vi "Scan start (SubVI).vi"(0 "VISA Refnum in":refnum<visa-resource-name>="COM7", 1 "end_x":dbl, 2 "end_y":dbl, 3 "sp_x":dbl, 4 "sp_y":dbl, 5 "error in":errorcluster, 8 "Режим\nсканирования":enum32{"Ampl", "Phase"}(ring), 9 "step_x":u32, 10 "pos_xy":cluster{"pos_x":dbl, "pos_y":dbl} caption="Позиция 2D, мм", 11 "step_y":u32) -> (14 "VISA resource name out":refnum<visa-resource-name>, 16 "set_pos_xy":cluster{"pos_x":dbl, "pos_y":dbl} caption="Set pos 2D, мм", 19 "error out":errorcluster)   [LabVIEW 2018]
uses:
  GlobalStop.vi
panel:
  out "err":errorcluster
  in  "Average":u8=5 caption="Число усреднений\nАЦП" min=1 max=9
  in  "Smooth":bool=TRUE caption="Аппроксимировать\nзначения с АЦП"
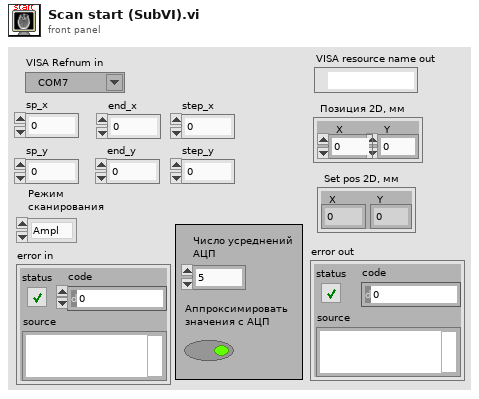
[diagram p1: front panel]
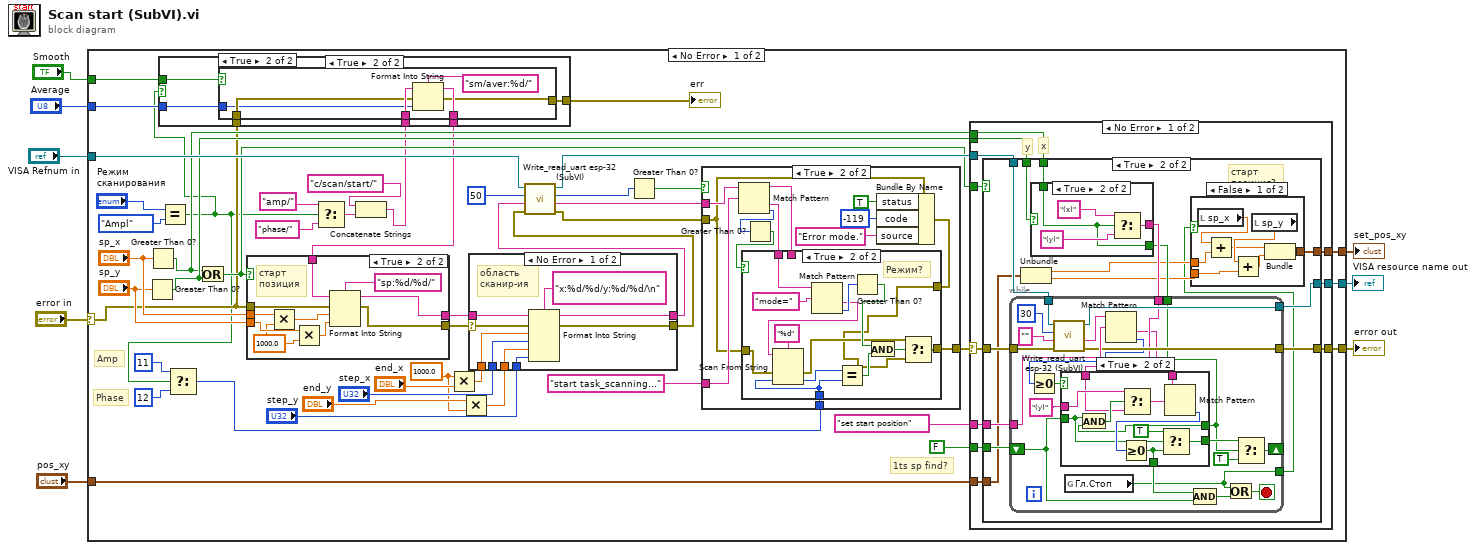
[diagram p0: block diagram]
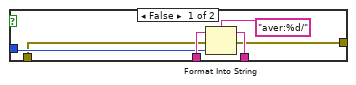
[diagram p3: hidden frame]
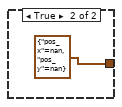
[diagram p5: hidden frame]
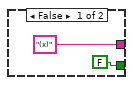
[diagram p6: hidden frame]
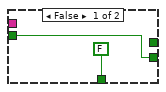
[diagram p7: hidden frame]
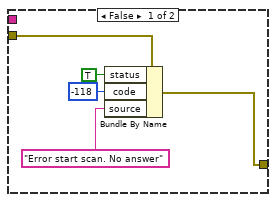
[diagram p9: hidden frame]
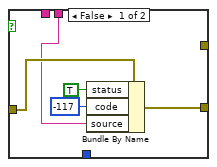
[diagram p10: hidden frame]
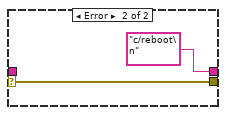
[diagram p11: hidden frame]
diagram:
  n1 = case shown="No Error" "error in" {
    selector: "error in" -> [w11 w219]
    tunnel: [w24 w219] -> w7
    tunnel: [w26 w218] -> w6
    tunnel: "VISA Refnum in" -> [w25 w218]
    tunnel: "pos_xy" -> [w17 w217]
    tunnel: [w16 w217] -> w3
    tunnel: "Smooth" -> [w15 _]
    tunnel: "Average" -> [w12 _]
    frame No Error {
      w29 = 1000.0
      # "1ts sp find?"
      # "Phase"
      # "Amp"
      n2 = Greater Than 0?(x="sp_y") -> (x > 0?=w21:bool)
      n3 = Greater Than 0?(x="sp_x") -> (x > 0?=w20:bool)
      n4 = Equal?(x="Режим\nсканирования", y=enum32{"Ampl", "Phase"}."Ampl") -> (x = y?=w9:bool)
      n5 = Select(t=u8 11, s=w9, f=u8 12) -> (s? t:f=w33:u8)
      n6 = Or(x=w20, y=w21) -> (x .or. y?=w23:bool)
      n7 = Select(t="amp/" ("initial string"), s=w9, f="phase/" ("initial string")) -> (s? t:f=w54:string)
      n8 = Concatenate Strings("c/scan/start/" ("initial string"), w54) -> (w14:string)
      n9 = case shown="True" w9 {
        tunnel: w15 -> [_ w63]
        tunnel: w14 -> [w57 w62]
        tunnel: [w57 w61] -> w13
        tunnel: w12 -> [_ w60]
        tunnel: w11 -> [w56 w59]
        tunnel: [w56 w58] -> w10
        frame False {
        }
        frame True {
          n10 = case shown="True" w63 {
            tunnel: w62 -> [w69 w73]
            tunnel: [w68 w74] -> w61
            tunnel: w60 -> [w66 w71]
            tunnel: w59 -> [w65 w72]
            tunnel: [w64 w70] -> w58
            frame False {
              n11 = Format Into String(format string="aver:%d/" ("initial string"), initial string=w69, error in=w65, w66) -> (resulting string=w68:string, error out=w64:errorcluster)
            }
            frame True {
              n12 = Format Into String(format string="sm/aver:%d/" ("initial string"), initial string=w73, error in=w72, w71) -> (resulting string=w74:string, error out=w70:errorcluster)
            }
          }
        }
      }
      "err" <- w10
      n13 = case shown="True" w23 {
        tunnel: w13 -> [w205 w216]
        tunnel: "sp_x" -> [_ w210]
        tunnel: "sp_y" -> [_ w211]
        tunnel: w11 -> [w206 w214]
        tunnel: [w206 w212] -> w47
        tunnel: [w205 w213] -> w46
        frame False {
        }
        frame True {
          w209 = 1000.0
          # "старт\nпозиция"
          n14 = Multiply(x=w210, y=w209) -> (x*y=w207:dbl)
          n15 = Multiply(x=w211, y=w209) -> (x*y=w208:dbl)
          n16 = Format Into String(format string="sp:%d/%d/", initial string=w216, error in=w214, w207, w208) -> (resulting string=w213:string, error out=w212:errorcluster)
        }
      }
      n17 = Multiply(x=w29, y="end_x") -> (x*y=w31:dbl)
      n18 = Multiply(x="end_y", y=w29) -> (x*y=w28:dbl)
      n19 = case shown="No Error" w47 {
        selector: w47 -> [w201 w204]
        tunnel: w46 -> [w202 _]
        tunnel: w31 -> [w200 _]
        tunnel: "step_x" -> [w198 _]
        tunnel: w28 -> [w197 _]
        tunnel: "step_y" -> [w196 _]
        tunnel: [w195 w204] -> w42
        tunnel: [w194 "c/reboot\n"] -> w41
        frame No Error {
          # "область\nсканир-ия"
          n20 = Format Into String(format string="x:%d/%d/y:%d/%d/\n", initial string=w202, error in=w201, w200, w198, w197, w196) -> (resulting string=w194:string, error out=w195:errorcluster)
        }
        frame Error {
        }
      }
      n21 = call "Write_read_uart esp-32 (SubVI).vi"("error in (no error)"=w42, "write buffer"=w41, "milliseconds to wait"=u32 50, "VISA Refnum in"=w25) -> ("error out 4"=w37:errorcluster, "read buffer"=w40:string, "read bite"=w39:u32, "VISA resource name out"=w27:refnum<visa-resource-name>)
      n22 = Greater Than 0?(x=w39) -> (x > 0?=w38:bool)
      n23 = case shown="True" w38 {
        tunnel: w40 -> [_ w174]
        tunnel: w37 -> [w159 w166]
        tunnel: "start task_scanning..." -> [_ w173]
        tunnel: w33 -> [_ w169]
        tunnel: [w158 w164] -> w18
        frame False {
          n24 = Bundle By Name(cluster=w159, "status"=TRUE, "code"=i16 -118, "source"="Error start scan. No answer") -> (w158:errorcluster)
        }
        frame True {
          n25 = Match Pattern(string=w174, regular expression=w173) -> (before substring=w162:string, after substring=w170:string, offset past match=w172:i32)  [unwired: 1 in, 1 out]
          n26 = Greater Than 0?(x=w172) -> (x > 0?=w171:bool)
          n27 = Bundle By Name(cluster=w166, "status"=TRUE, "code"=i16 -119, "source"="Error mode.") -> (w165:errorcluster)
          n28 = case shown="True" w171 {
            tunnel: w170 -> [_ w193]
            tunnel: w166 -> [w178 w188]
            tunnel: w169 -> [_ w187]
            tunnel: w165 -> [_ w181]
            tunnel: [w177 w180] -> w164
            tunnel: w162 -> [w175 _]
            frame False {
              n29 = Bundle By Name(cluster=w178, "status"=TRUE, "code"=i16 -117, "source"=w175) -> (w177:errorcluster)
            }
            frame True {
              # "Режим?"
              n30 = Match Pattern(string=w193, regular expression="mode=") -> (after substring=w189:string, offset past match=w191:i32)  [unwired: 1 in, 2 out]
              n31 = Scan From String(format string="%d", input string=w189, error in=w188, default 1=w187) -> (error out=w182:errorcluster, output 1=w186:u8)  [unwired: 1 in, 2 out]
              n32 = Equal?(x=w186, y=w187) -> (x = y?=w184:bool)
              n33 = Greater Than 0?(x=w191) -> (x > 0?=w185:bool)
              n34 = And(x=w185, y=w184) -> (x .and. y?=w183:bool)
              n35 = Select(t=w182, s=w183, f=w181) -> (s? t:f=w180:errorcluster)
            }
          }
        }
      }
      n36 = case shown="No Error" w18 {
        selector: w18 -> [w78 w155]
        tunnel: w27 -> [w86 w156]
        tunnel: [w85 w156] -> w26
        tunnel: [w84 w155] -> w24
        tunnel: w23 -> [w83 _]
        tunnel: "set start position" -> [w82 _]
        tunnel: w21 -> [w81 _]
        tunnel: w20 -> [w80 _]
        tunnel: FALSE -> [w79 _]
        tunnel: w17 -> [w77 w154]
        tunnel: [w76 w154] -> w16
        frame No Error {
          # "x"
          # "y"
          n37 = case shown="True" w83 {
            tunnel: w86 -> [w89 w104]
            tunnel: [w89 w103] -> w85
            tunnel: w78 -> [w88 w102]
            tunnel: [w88 w101] -> w84
            tunnel: w82 -> [_ w100]
            tunnel: w81 -> [_ w99]
            tunnel: w80 -> [_ w98]
            tunnel: w79 -> [_ w96]
            tunnel: w77 -> [w87 w94]
            tunnel: [w87 w90] -> w76
            frame False {
            }
            frame True {
              # "старт\nпозиция?"
              n38 = Unbundle(w94) -> ("pos_x"=w93:dbl, "pos_y"=w92:dbl)
              n39 = case shown="True" w99 {
                tunnel: w98 -> [_ w115]
                tunnel: ["(x)" w116] -> w97
                tunnel: [FALSE w115] -> w95
                frame False {
                }
                frame True {
                  n40 = Select(t="(x)", s=w115, f="(y)") -> (s? t:f=w116:string)
                }
              }
              n41 = while {
                tunnel: w104 -> [w140]
                tunnel: [w139] -> w103
                tunnel: w102 -> [w136]
                tunnel: [w133] -> w101
                tunnel: w100 -> [w134]
                tunnel: w97 -> [w124]
                shift-right: [w129] -> _
                shift-left: w96 -> [w128]
                tunnel: w95 -> [w120]
                tunnel: [w121] -> w91
                stop <- w122 stop-if-true
                n42 = call "Write_read_uart esp-32 (SubVI).vi"("error in (no error)"=w136, "write buffer"="", "milliseconds to wait"=u32 30, "VISA Refnum in"=w140) -> ("error out 4"=w133:errorcluster, "read buffer"=w135:string, "VISA resource name out"=w139:refnum<visa-resource-name>)  [unwired: 1 out]
                n43 = global read "GlobalStop.vi" "Гл.Стоп"() -> (w121:bool)
                n44 = Match Pattern(string=w135, regular expression=w134) -> (after substring=w119:string, offset past match=w131:i32)  [unwired: 1 in, 2 out]
                n45 = Greater Or Equal To 0?(x=w131) -> (x >= 0?=w132:bool)
                n46 = case shown="True" w132 {
                  tunnel: w119 -> [_ w153]
                  tunnel: [w142 w149] -> w130
                  tunnel: w128 -> [w142 w146]
                  tunnel: "(y)" -> [_ w151]
                  tunnel: [FALSE w147] -> w125
                  tunnel: w124 -> [_ w144]
                  tunnel: w120 -> [_ w143]
                  frame False {
                  }
                  frame True {
                    n47 = And(x=w146, y=w143) -> (x .and. y?=w145:bool)
                    n48 = Select(t=w151, s=w145, f=w144) -> (s? t:f=w150:string)
                    n49 = Match Pattern(string=w153, regular expression=w150) -> (offset past match=w152:i32)  [unwired: 1 in, 3 out]
                    n50 = Greater Or Equal To 0?(x=w152) -> (x >= 0?=w147:bool)
                    n51 = Select(t=TRUE, s=w146, f=w147) -> (s? t:f=w149:bool)
                  }
                }
                n52 = Compound Arithmetic op=AND(w125, w128) -> (w123:bool)
                n53 = Or(x=w121, y=w123) -> (x .or. y?=w122:bool)
                n54 = Select(t=w130, s=w120, f=TRUE ("t")) -> (s? t:f=w129:bool)
              }
              n55 = case shown="False" w91 {
                tunnel: w93 -> [w111 _]
                tunnel: w92 -> [w109 _]
                tunnel: [w105 cluster{"pos_x":dbl, "pos_y":dbl} {"pos_x"=nan, "pos_y"=nan} ("pos_xy")] -> w90
                frame False {
                  n56 = local read "sp_x"() -> (w110:dbl)
                  n57 = Add(x=w110, y=w111) -> (x+y=w106:dbl)
                  n58 = local read "sp_y"() -> (w108:dbl)
                  n59 = Add(x=w108, y=w109) -> (x+y=w107:dbl)
                  n60 = Bundle(w106, w107) -> (w105:cluster{dbl, dbl})  [unwired: 1 in]
                }
                frame True {
                }
              }
            }
          }
        }
        frame Error {
        }
      }
    }
    frame Error {
    }
  }
  "error out" <- w7
  "VISA resource name out" <- w6
  "set_pos_xy" <- w3
